vi "2D String Array_DeleteSelectedCells.vi"(10 "Indexes":i32[](array[numeric]), 11 "2D Array.In":string[][](array[string])) -> (3 "2D Array.Out":string[][](array[string]))   [LabVIEW 2024]
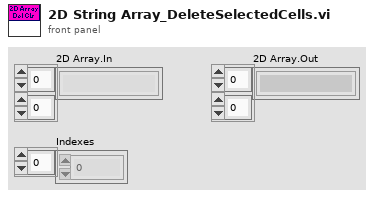
[diagram p1: front panel]
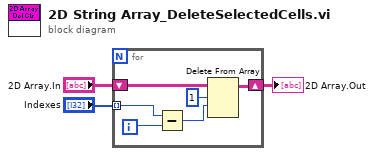
[diagram p0: block diagram]
diagram:
  n1 = for {
    shift-right: [w7] -> w3
    shift-left: "2D Array.In" -> [w9]
    tunnel: "Indexes" -> [w5] mode=indexing
    i -> [w6]
    n2 = Subtract(x=w5, y=w6) -> (x-y=w4:i32)
    n3 = Delete From Array(array=w9, length=1, index (row)=w4) -> (array with subset deleted=w7:string[][])  [unwired: 1 in, 1 out]
  }
  "2D Array.Out" <- w3
